vi "Screen_Traduction.vi"() -> ()   [LabVIEW 2013]
uses:
  030 - EVENTS/EnumFgvEventCommand.ctl
  ContexteTraduction.ctl
  080 - TOOLS/Traduction/Dictionnary/Dictionnaire.ctl
  080 - TOOLS/Traduction/Dictionnary/CleValeur.ctl
  090 - ERRORS/Ctrls/enumLogAndView.ctl
  080 - TOOLS/Traduction/Dictionnary/EnumCommandDictionnaire.ctl
  <vilib>/Utility/miscctls.llb/LVComboBoxStrsAndValuesArrayTypeDef.ctl
  050 - CONFIG/00 - ApplicationConfig/Ctrls/EnumFgvConfigCommand.ctl
  enumScreen.ctl
panel:
  in  "Dictionnaire":string(combo)
  in  "Supprimer Dictionnaire":bool
  in  "Dupliquer Dictionnaire":bool
  in  "Dictionnaire verrouillé ?":bool
  in  "Clés":i32[](listbox)
  in  "Supprimer Lignes":bool
  out "Valeur de référence":string
  in  "Valeur traduite":string
  in  "Bouton menu principal":bool
  # "Attention : Si la \"valeur traduite\" contient des caractères de type %s, %d, %f ..., il s'agit de caractères de formattage\nde messages dynamiques. Il faut absolument que ces caractères apparaîssent dans la chaîne modifiée, et dans\nle même ordre.\nPour info : %s remplace une chaîne de caractères, %d remplace un entier, %f remplace un nombre à virgules \nflottantes. (Voir syntaxe du langage C)"
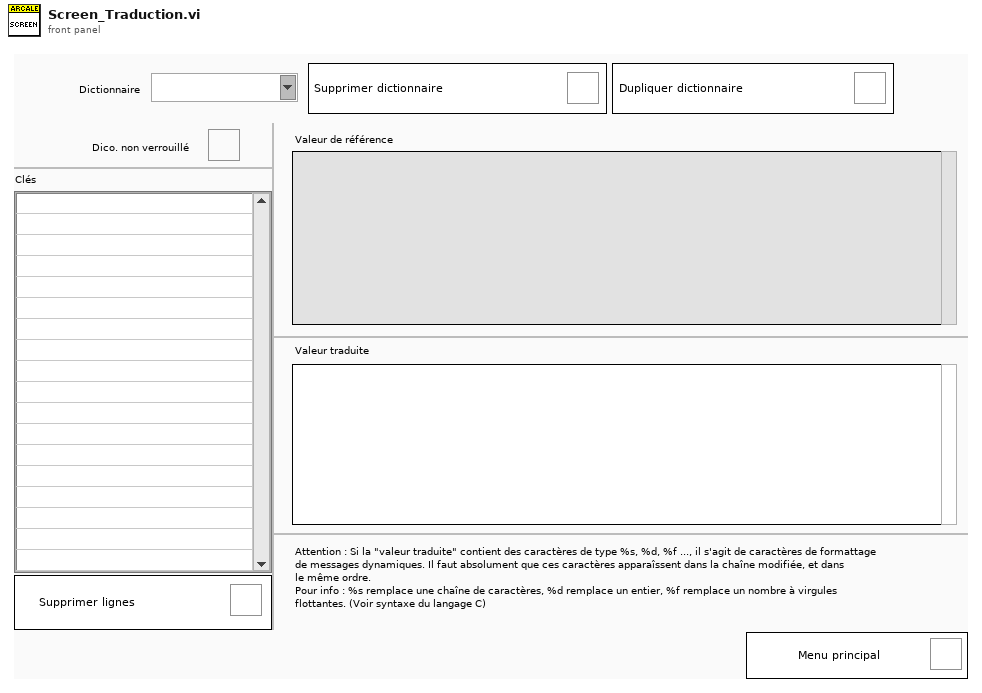
[diagram p1: front panel]
types:
  T1 = typedef "enumLogAndView.ctl" = enum16{"Log only", "Log and view"}
  T2 = typedef "ContexteTraduction.ctl" = cluster{"Dictionnaire":T3}
  T3 = typedef "Dictionnaire.ctl" = cluster{"FichierDictionnaire":path, "TabCleValeur":T4[], "DictionnaireModifié?":bool, "Traduction à réaliser ?":bool, "Interdire l'ajout de nouvelles clés ?":bool}
  T4 = typedef "CleValeur.ctl" = cluster{"Clé":string, "Valeur":string}
  T5 = typedef "EnumFgvEventCommand.ctl" = enum16{"Setup", "Cleanup", "Get"}
  T6 = typedef "EnumFgvConfigCommand.ctl" = enum16{"Load", "Get", "Set", "Save To Disk"}
  T7 = typedef "LVComboBoxStrsAndValuesArrayTypeDef.ctl" = cluster{"String":string, "Value":string}[]
  T8 = typedef "EnumCommandDictionnaire.ctl" = enum16{"Load", "Translate", "Save", "GetDico", "Set : A traduire = Vrai", "Set : A Traduire = Faux", "SetDico"}
  T9 = typedef "ApplicationConfig.ctl" = cluster{"Data Path":path, "MessageHandlerConfig":T10, "Simulation":bool, "Dictionnary":string}
  T10 = typedef "MessageHandlerConfig.ctl" = cluster{"Max log files":u32, "Max messages per file":u32}
  T11 = enum8{"Enabled", "Disabled", "Disabled and Grayed Out"}
  T12 = typedef "enumScreen.ctl" = enum16{"Test screen", "Ecran principal", "LOG", "Setup", "Popup : About", "Popup : View last message", "Popup : WebBrowser help", "Traduction", "Popup : DEBUG Process"}
  T13 = typedef "ToScreensCommand.ctl" = enum16{"Stop screen", "Stop all screens"}
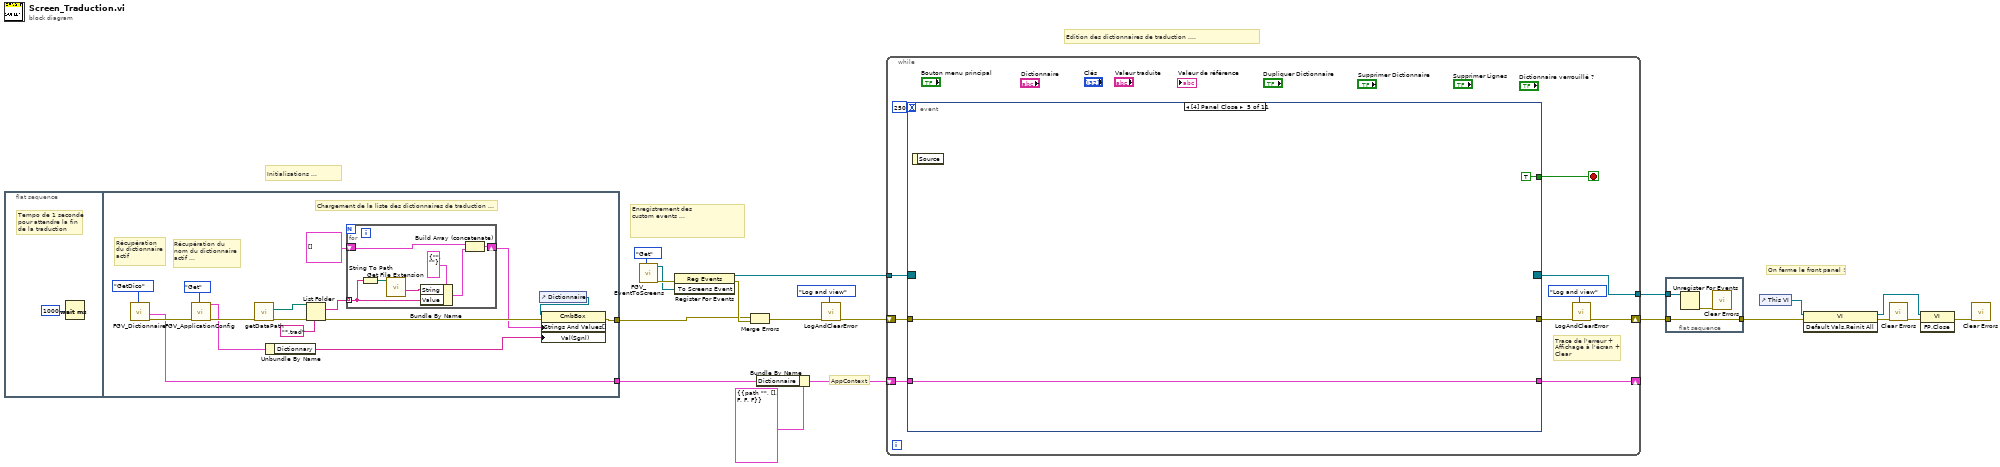
[diagram p0: block diagram]
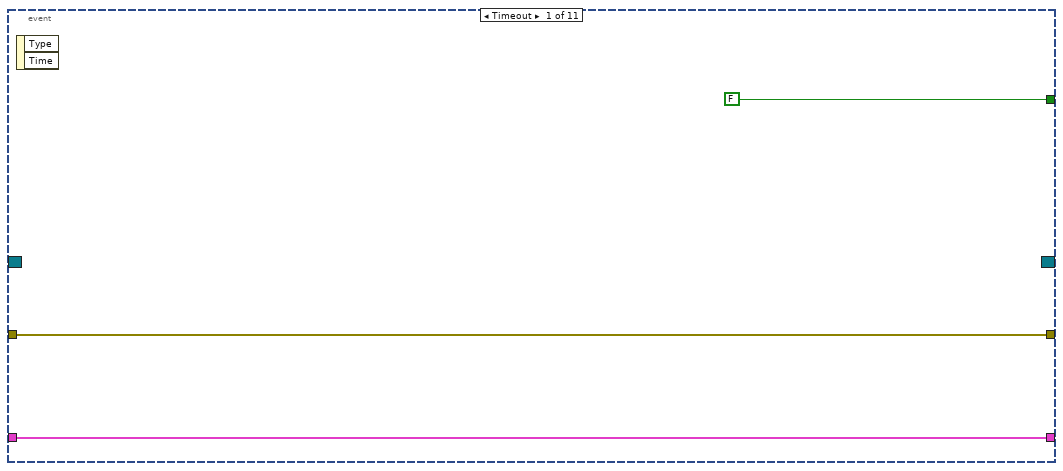
[diagram p2: hidden frame]
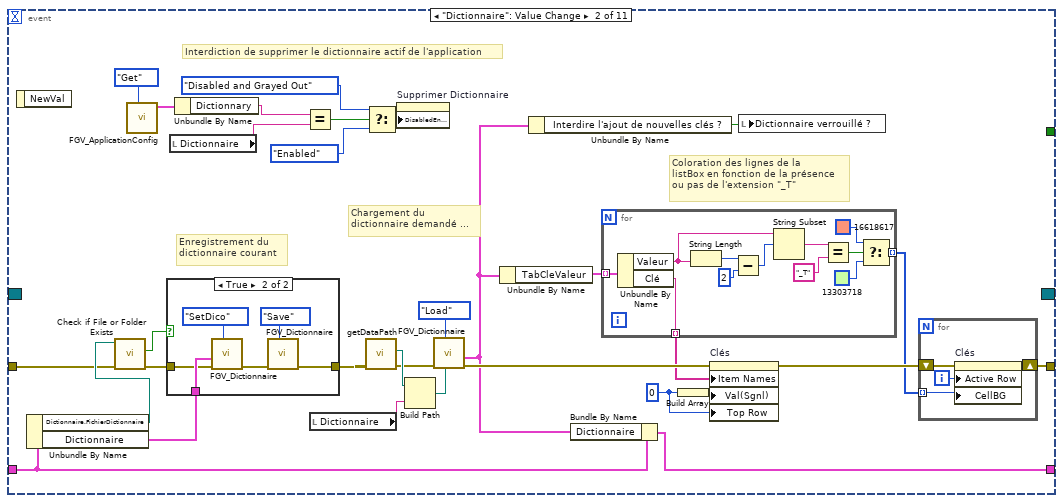
[diagram p3: hidden frame]
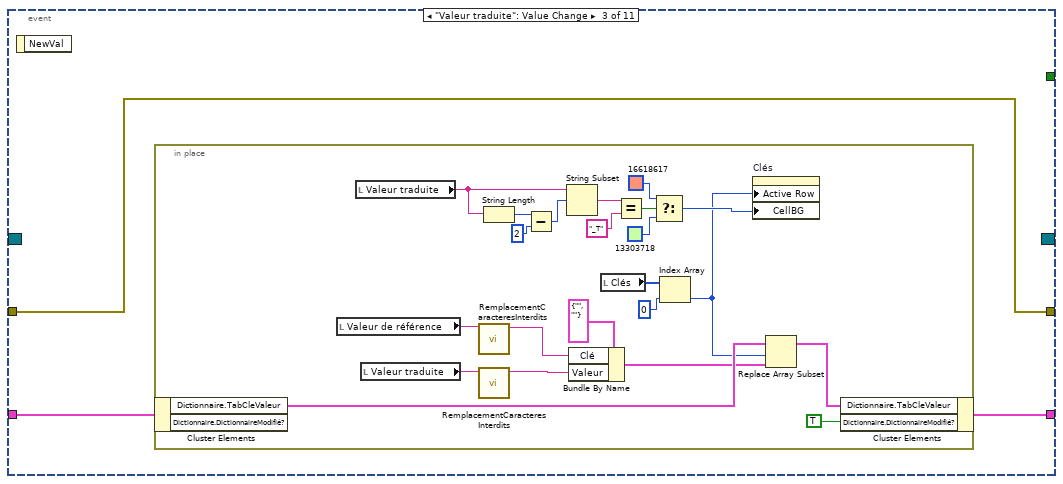
[diagram p5: hidden frame]
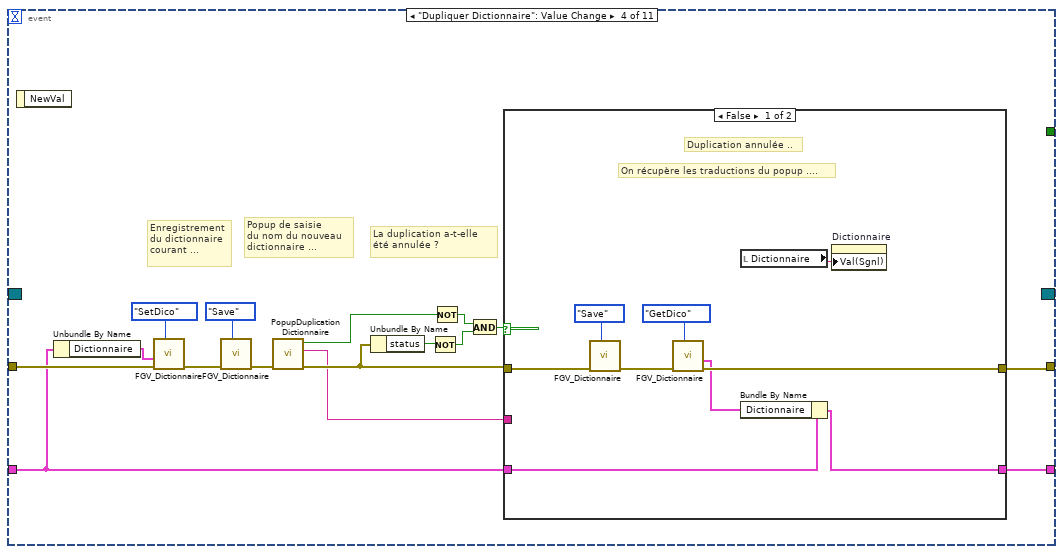
[diagram p6: hidden frame]
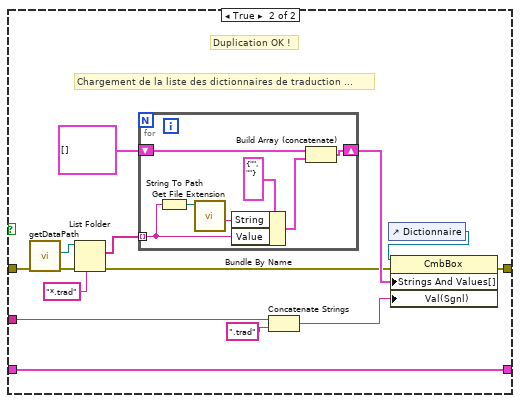
[diagram p7: hidden frame]
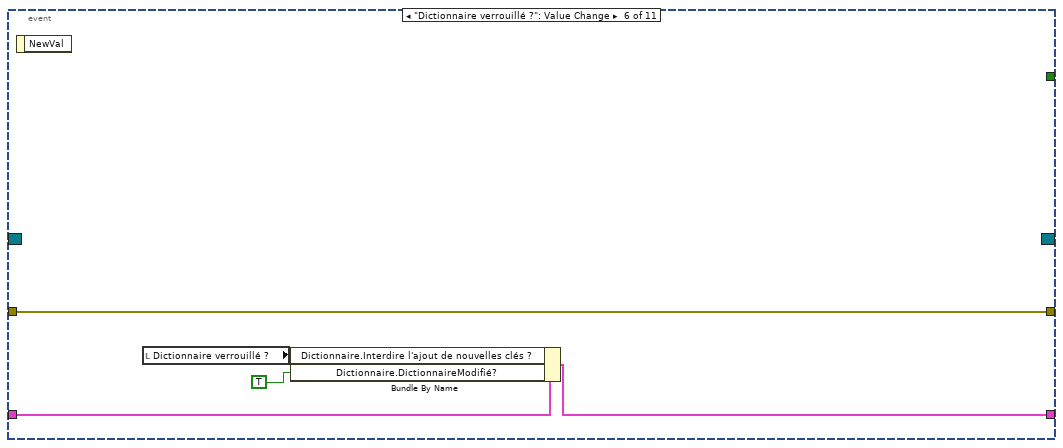
[diagram p8: hidden frame]
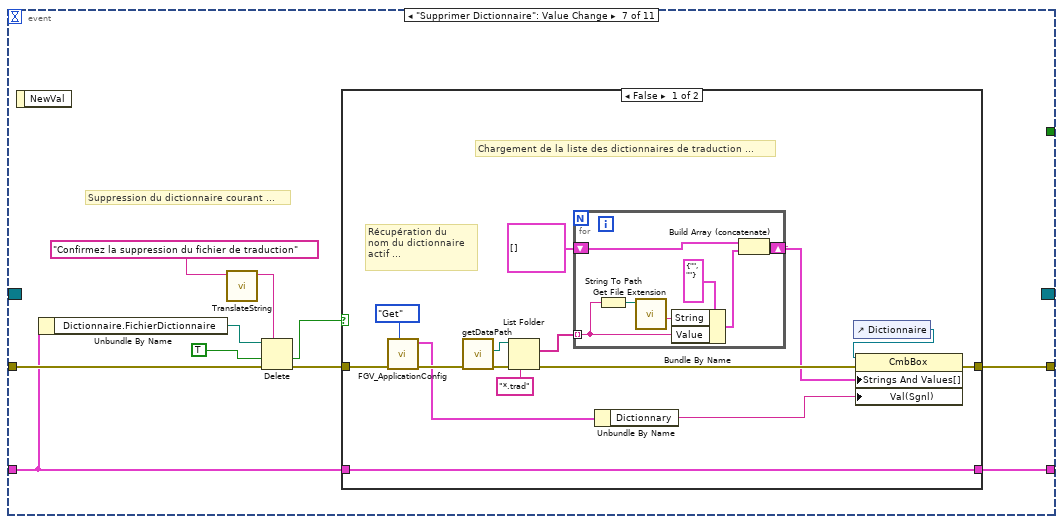
[diagram p9: hidden frame]
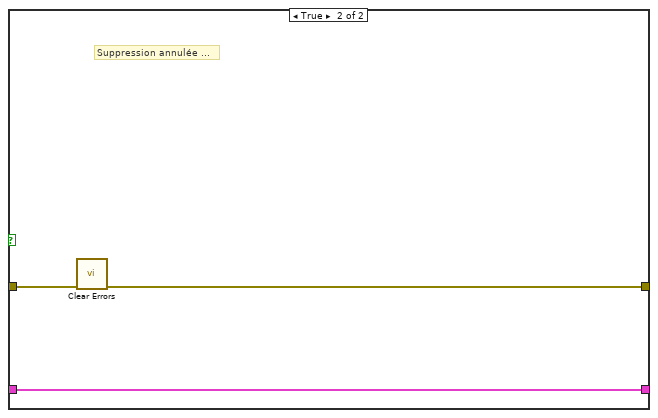
[diagram p10: hidden frame]
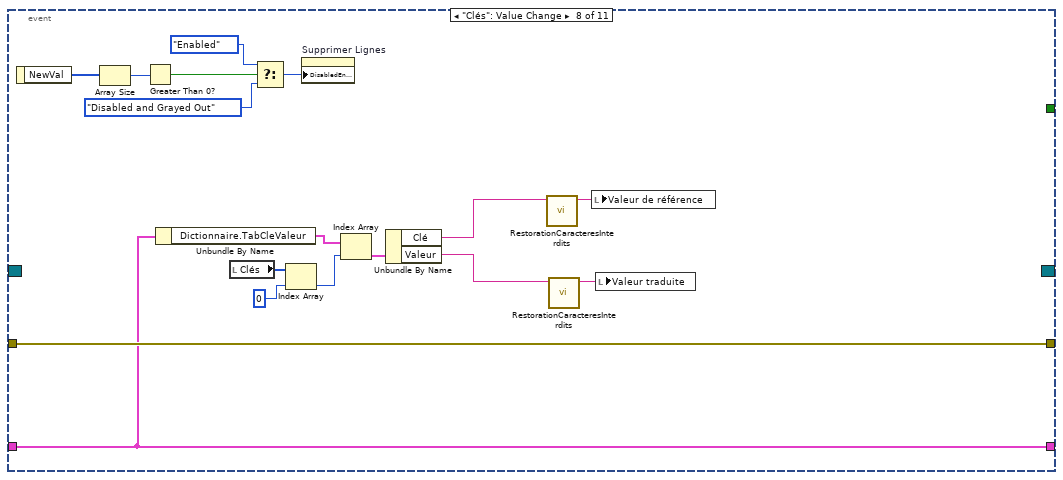
[diagram p11: hidden frame]
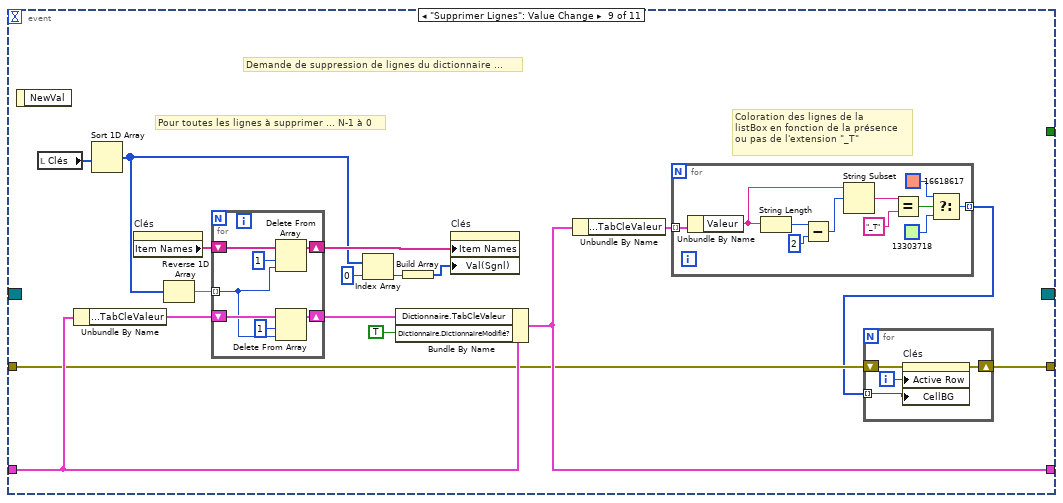
[diagram p12: hidden frame]
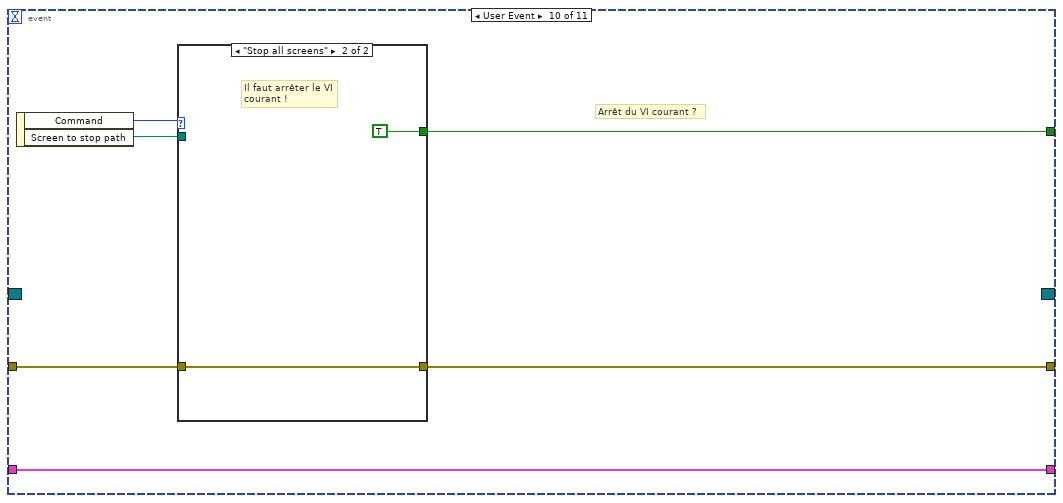
[diagram p13: hidden frame]
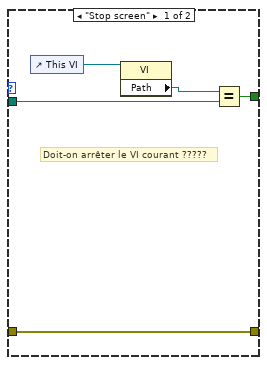
[diagram p14: hidden frame]
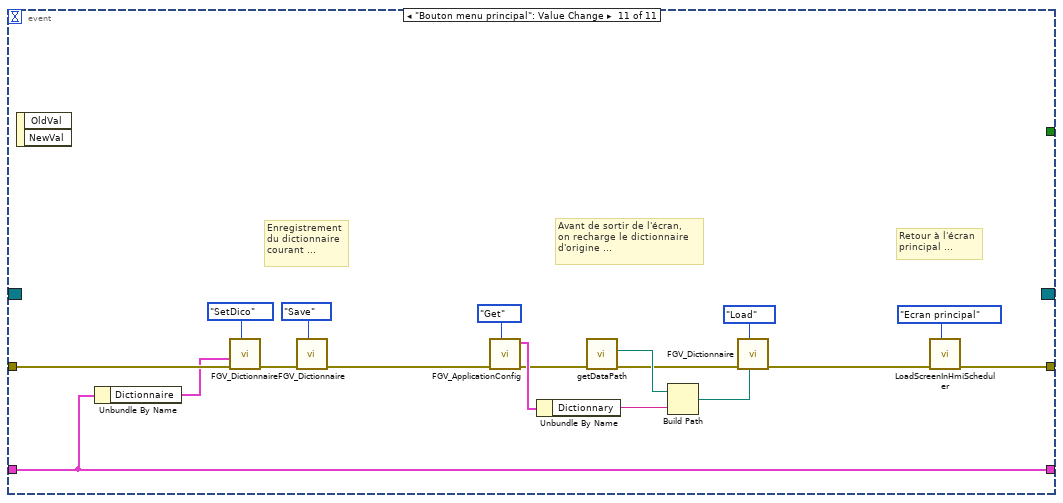
[diagram p15: hidden frame]
diagram:
  # "AppContext"
  # "Enregistrement des\ncustom events ..."
  # "Initialisations ..."
  # "On ferme le front panel !"
  # "Edition des dictionnaires de traduction ...."
  n1 = flat-sequence {
    tunnel: [w29] -> w9
    tunnel: [w22] -> w7
    frame #0 {
      # "Tempo de 1 seconde\npour attendre la fin\nde la traduction"
      n2 = Wait (ms)(milliseconds to wait=u32 1000) -> ()  [unwired: 1 out]
    }
    frame #1 {
      # "Récupération du\nnom du dictionnaire\nactif ..."
      # "Chargement de la liste des dictionnaires de traduction ..."
      # "Récupération \ndu dictionnaire\nactif"
      n3 = call "FGV_Dictionnaire.vi"("Command"=EnumCommandDictionnaire."GetDico") -> ("error out"=w28:errorcluster, "Dictionnaire Out"=w22:T3)  [unwired: 8 in, 1 out]
      n4 = call "FGV_ApplicationConfig.vi"("Command"=EnumFgvConfigCommand."Get", "error in (no error)"=w28) -> ("error out"=w27:errorcluster, "ApplicationConfigOut"=w25:T9)  [unwired: 8 in]
      n5 = call "getDataPath.vi"("error in (no error)"=w27) -> ("error out"=w32:errorcluster, "DataPath"=w36:path)  [unwired: 9 in]
      n6 = Unbundle By Name(w25) -> ("Dictionnary"=w24:string)
      n7 = List Folder(path=w36, pattern="*.trad", error in=w32) -> (filenames=w34:string[], error out=w31:errorcluster)  [unwired: 1 in, 2 out]
      n8 = for {
        tunnel: w34 -> [w40] mode=indexing
        shift-right: [w43] -> w23
        shift-left: T7 [] ("Strings And Values []") -> [w44]
        n9 = String To Path(string=w40) -> (path=w39:path)
        n10 = call <vilib>:"Get File Extension.vi"("file"=w39) -> ("filename without extension"=w38:string)  [unwired: 7 in, 3 out]
        n11 = Bundle By Name(cluster=cluster{"String":string, "Value":string} {"String"="", "Value"=""}, "String"=w38, "Value"=w40) -> (w41:cluster{"String":string, "Value":string})
        n12 = Build Array (concatenate)(w44, w41) -> (w43:T7)
      }
      n13 = control-ref of="Dictionnaire"() -> (w30:refnum<vi>)
      n14 = property on="Property Node" class="CmbBox"(reference=w30, error in=w31, "Strings And Values[]"=w23, "Val(Sgnl)"=w24) -> (error out=w29:errorcluster)  [unwired: 1 out]
    }
  }
  n15 = call "FGV_EventToScreens.vi"("Command"=EnumFgvEventCommand."Get") -> ("error out"=w20:errorcluster, "To Screens Event"=w19:refnum<user-event>)  [unwired: 9 in]
  n16 = register-events(error in=w20, w19) -> (reference out=w18:refnum<event-registration>, error out=w11:errorcluster)  [unwired: 1 in]
  n17 = Merge Errors(w9, w11) -> (w5:errorcluster)
  n18 = Bundle By Name(cluster=T2 {"Dictionnaire"={"FichierDictionnaire"=path "", "TabCleValeur"=[], "DictionnaireModifié?"=FALSE, "Traduction à réaliser ?"=FALSE, "Interdire l'ajout de nouvelles clés ?"=FALSE}} ("Contexte"), "Dictionnaire"=w7) -> (w8:T2)
  n19 = call "LogAndClearError.vi"("Log and view ?"=enumLogAndView."Log and view", "error in (no error)"=w5) -> ("error out"=w4:errorcluster)  [unwired: 9 in]
  n20 = while {
    tunnel: w18 -> [w54]
    shift-right: [w48] -> w16
    shift-left: w4 -> [w53]
    tunnel: [w52] -> w17
    shift-right: [w49] -> _
    shift-left: w8 -> [w50]
    stop <- w51 stop-if-true
    # "Trace de l'erreur +\nAffichage à l'écran +\nClear"
    n21 = event shown="[4] Panel Close" {
      selector: w54 -> [_ _ _ _ _ _ _ _ _ _ _]
      dyn-events: [_ _ _ _ _ _ _ _ _ _ _] -> w52
      timeout: 250 -> [_ _ _ _ _ _ _ _ _ _ _]
      tunnel: w53 -> [w57 w68 w112 w149 w185 w190 w200 w240 w245 w286 w298]
      tunnel: [w57 w78 w112 w140 w185 w190 w192 w240 w244 w285 w311] -> w47
      tunnel: [FALSE _ _ _ TRUE _ _ _ _ w283 _] -> w51
      tunnel: w50 -> [w55 w75 w114 w138 w184 w189 w193 w239 w256 w282 w296]
      tunnel: [w55 w82 w113 w137 w184 w188 w191 w239 w246 w282 w296] -> w49
      event Timeout {
        n22 = event-data() -> ()  [unwired: 1 in, 2 out]
      }
      event "Dictionnaire": Value Change {
        w71 = 0 ("Value (Signaling)")
        # "Interdiction de supprimer le dictionnaire actif de l'application"
        # "Coloration des lignes de la\nlistBox en fonction de la présence\nou pas de l'extension \"_T\""
        # "Enregistrement du\ndictionnaire courant"
        # "Chargement du \ndictionnaire demandé ..."
        n23 = event-data() -> ()  [unwired: 1 in, 1 out]
        n24 = Unbundle By Name(w75) -> ("Dictionnaire.FichierDictionnaire"=w73:path, "Dictionnaire"=w76:T3)
        n25 = call <vilib>:"Check if File or Folder Exists.vi"("error in (no error)"=w68, "path"=w73) -> ("error out"=w74:errorcluster, "file or folder exists?"=w72:bool)  [unwired: 7 in, 1 out]
        n26 = call "FGV_ApplicationConfig.vi"("Command"=EnumFgvConfigCommand."Get") -> ("ApplicationConfigOut"=w66:T9)  [unwired: 9 in, 1 out]
        n27 = case shown="True" w72 {
          tunnel: [w89 w94] -> w81
          tunnel: w76 -> [_ w91]
          tunnel: w74 -> [w89 w90]
          frame False {
          }
          frame True {
            n28 = call "FGV_Dictionnaire.vi"("Command"=EnumCommandDictionnaire."SetDico", "error in (no error)"=w90, "Dictionnaire In"=w91) -> ("error out"=w92:errorcluster)  [unwired: 6 in, 2 out]
            n29 = call "FGV_Dictionnaire.vi"("Command"=EnumCommandDictionnaire."Save", "error in (no error)"=w92) -> ("error out"=w94:errorcluster)  [unwired: 7 in, 2 out]
          }
        }
        n30 = local read "Dictionnaire"() -> (w65:string)
        n31 = Unbundle By Name(w66) -> ("Dictionnary"=w64:string)
        n32 = Equal?(x=w64, y=w65) -> (x = y?=w61:bool)
        n33 = local read "Dictionnaire"() -> (w77:string)
        n34 = call "getDataPath.vi"("error in (no error)"=w81) -> ("error out"=w86:errorcluster, "DataPath"=w88:path)  [unwired: 9 in]
        n35 = Select(t=T11."Disabled and Grayed Out" ("Disabled"), s=w61, f=T11."Enabled" ("Disabled")) -> (s? t:f=w63:T11)
        n36 = property on="Supprimer Dictionnaire" class="Bool"("DisabledEnum"=w63) -> ()  [unwired: 2 in, 2 out]
        n37 = Build Path(base path=w88, name or relative path=w77) -> (appended path=w85:path)
        n38 = call "FGV_Dictionnaire.vi"("FichierDictionnaire"=w85, "Command"=EnumCommandDictionnaire."Load", "error in (no error)"=w86) -> ("error out"=w84:errorcluster, "Dictionnaire Out"=w59:T3)  [unwired: 6 in, 1 out]
        n39 = Unbundle By Name(w59) -> ("TabCleValeur"=w69:T4[])
        n40 = Unbundle By Name(w59) -> ("Interdire l'ajout de nouvelles clés ?"=w58:bool)
        n41 = Bundle By Name(cluster=w75, "Dictionnaire"=w59) -> (w82:T2)
        n42 = for {
          tunnel: w69 -> [w111] mode=indexing
          tunnel: [w110] -> w83 mode=indexing
          tunnel: [w100] -> w79 mode=indexing
          n43 = Unbundle By Name(w111) -> ("Valeur"=w109:string, "Clé"=w110:string)
          n44 = String Length(string=w109) -> (length=w108:i32)
          n45 = Subtract(x=w108, y=2) -> (x-y=w106:i32)
          n46 = String Subset(string=w109, offset (0)=w106) -> (substring=w105:string)  [unwired: 1 in]
          n47 = Equal?(x=w105, y="_T") -> (x = y?=w103:bool)
          n48 = Select(t=u32 16618617, s=w103, f=u32 13303718) -> (s? t:f=w100:u32)
        }
        n49 = Build Array(w71) -> (w70:i32[])
        n50 = property on="Clés" class="LstBox (strict)"(error in=w84, "Item Names"=w83, "Val(Sgnl)"=w70, "Top Row"=w71) -> (error out=w80:errorcluster)  [unwired: 1 in, 1 out]
        n51 = local write "Dictionnaire verrouillé ?"(w58) -> ()
        n52 = for {
          shift-right: [w98] -> w78
          shift-left: w80 -> [w99]
          tunnel: w79 -> [w97] mode=indexing
          i -> [w96]
          n53 = property on="Clés" class="LstBox (strict)"(error in=w99, "Active Row"=w96, "CellBG"=w97) -> (error out=w98:errorcluster)  [unwired: 1 in, 1 out]
        }
      }
      event "Valeur traduite": Value Change {
        n54 = event-data() -> ()  [unwired: 1 in, 1 out]
        n55 = in-place {
          n56 = in-place-cluster #1(w114) -> ("Dictionnaire.TabCleValeur"=w135:T4[])  [unwired: 1 out]
          n57 = local read "Valeur de référence"() -> (w121:string)
          n58 = local read "Valeur traduite"() -> (w123:string)
          n59 = local read "Valeur traduite"() -> (w119:string)
          n60 = call "RemplacementCaracteresInterdits.vi"("String In"=w121) -> ("String Out"=w120:string)  [unwired: 9 in, 1 out]
          n61 = call "RemplacementCaracteresInterdits.vi"("String In"=w119) -> ("String Out"=w118:string)  [unwired: 9 in, 1 out]
          n62 = String Length(string=w123) -> (length=w131:i32)
          n63 = Subtract(x=w131, y=2) -> (x-y=w129:i32)
          n64 = String Subset(string=w123, offset (0)=w129) -> (substring=w128:string)  [unwired: 1 in]
          n65 = Bundle By Name(cluster=T4 {"Clé"="", "Valeur"=""} ("new element/subarray"), "Clé"=w120, "Valeur"=w118) -> (w132:T4)
          n66 = local read "Clés"() -> (w117:i32[])
          n67 = Equal?(x=w128, y="_T") -> (x = y?=w126:bool)
          n68 = Select(t=u32 16618617, s=w126, f=u32 13303718) -> (s? t:f=w122:u32)
          n69 = Index Array(array=w117, index=0) -> (element=w115:i32)
          n70 = property on="Clés" class="LstBox (strict)"("Active Row"=w115, "CellBG"=w122) -> ()  [unwired: 2 in, 2 out]
          n71 = Replace Array Subset(array=w135, new element=w132, index=w115) -> (w134:T4[])
          n72 = in-place-cluster #1("Dictionnaire.TabCleValeur"=w134, "Dictionnaire.DictionnaireModifié?"=TRUE) -> (w113:T2)
        }
      }
      event "Dupliquer Dictionnaire": Value Change {
        # "La duplication a-t-elle\nété annulée ?"
        # "Popup de saisie\ndu nom du nouveau\ndictionnaire ..."
        # "Enregistrement\ndu dictionnaire\ncourant ..."
        n73 = event-data() -> ()  [unwired: 1 in, 1 out]
        n74 = Unbundle By Name(w138) -> ("Dictionnaire"=w147:T3)
        n75 = call "FGV_Dictionnaire.vi"("Command"=EnumCommandDictionnaire."SetDico", "error in (no error)"=w149, "Dictionnaire In"=w147) -> ("error out"=w150:errorcluster)  [unwired: 6 in, 2 out]
        n76 = call "FGV_Dictionnaire.vi"("Command"=EnumCommandDictionnaire."Save", "error in (no error)"=w150) -> ("error out"=w148:errorcluster)  [unwired: 7 in, 2 out]
        n77 = call "PopupDuplicationDictionnaire.vi"("error in (no error)"=w148) -> ("error out"=w141:errorcluster, "Nouveau dictionnaire Out"=w139:string, "Edition annulée ?"=w146:bool)  [unwired: 8 in]
        n78 = Unbundle By Name(w141) -> ("status"=w145:bool)
        n79 = Not(x=w145) -> (.not. x?=w143:bool)
        n80 = Not(x=w146) -> (.not. x?=w144:bool)
        n81 = And(x=w144, y=w143) -> (x .and. y?=w142:bool)
        n82 = case shown="False" w142 {
          tunnel: w141 -> [w160 w167]
          tunnel: [w157 w166] -> w140
          tunnel: w139 -> [_ w165]
          tunnel: w138 -> [w156 w162]
          tunnel: [w155 w162] -> w137
          frame False {
            # "On récupère les traductions du popup ...."
            # "Duplication annulée .."
            n83 = call "FGV_Dictionnaire.vi"("Command"=EnumCommandDictionnaire."Save", "error in (no error)"=w160) -> ("error out"=w158:errorcluster)  [unwired: 7 in, 2 out]
            n84 = call "FGV_Dictionnaire.vi"("Command"=EnumCommandDictionnaire."GetDico", "error in (no error)"=w158) -> ("error out"=w157:errorcluster, "Dictionnaire Out"=w154:T3)  [unwired: 7 in, 1 out]
            n85 = local read "Dictionnaire"() -> (w153:string)
            n86 = Bundle By Name(cluster=w156, "Dictionnaire"=w154) -> (w155:T2)
            n87 = property on="Dictionnaire" class="CmbBox"("Val(Sgnl)"=w153) -> ()  [unwired: 2 in, 2 out]
          }
          frame True {
            # "Chargement de la liste des dictionnaires de traduction ..."
            # "Duplication OK !"
            n88 = call "getDataPath.vi"("error in (no error)"=w167) -> ("error out"=w170:errorcluster, "DataPath"=w175:path)  [unwired: 9 in]
            n89 = List Folder(path=w175, pattern="*.trad", error in=w170) -> (filenames=w173:string[], error out=w169:errorcluster)  [unwired: 1 in, 2 out]
            n90 = for {
              tunnel: w173 -> [w176] mode=indexing
              shift-right: [w181] -> w171
              shift-left: T7 [] ("Strings And Values []") -> [w182]
              n91 = String To Path(string=w176) -> (path=w178:path)
              n92 = call <vilib>:"Get File Extension.vi"("file"=w178) -> ("filename without extension"=w177:string)  [unwired: 7 in, 3 out]
              n93 = Bundle By Name(cluster=cluster{"String":string, "Value":string} {"String"="", "Value"=""}, "String"=w177, "Value"=w176) -> (w179:cluster{"String":string, "Value":string})
              n94 = Build Array (concatenate)(w182, w179) -> (w181:T7)
            }
            n95 = Concatenate Strings(w165, ".trad" ("string")) -> (w164:string)
            n96 = control-ref of="Dictionnaire"() -> (w168:refnum<vi>)
            n97 = property on="Property Node" class="CmbBox"(reference=w168, error in=w169, "Strings And Values[]"=w171, "Val(Sgnl)"=w164) -> (error out=w166:errorcluster)  [unwired: 1 out]
          }
        }
      }
      event Panel Close {
        n98 = event-data() -> ()  [unwired: 1 in, 1 out]
      }
      event "Dictionnaire verrouillé ?": Value Change {
        n99 = event-data() -> ()  [unwired: 1 in, 1 out]
        n100 = local read "Dictionnaire verrouillé ?"() -> (w187:bool)
        n101 = Bundle By Name(cluster=w189, "Dictionnaire.Interdire l'ajout de nouvelles clés ?"=w187, "Dictionnaire.DictionnaireModifié?"=TRUE) -> (w188:T2)
      }
      event "Supprimer Dictionnaire": Value Change {
        # "Suppression du dictionnaire courant ..."
        n102 = event-data() -> ()  [unwired: 1 in, 1 out]
        n103 = Unbundle By Name(w193) -> ("Dictionnaire.FichierDictionnaire"=w199:path)
        n104 = call "TranslateString.vi"("String"="Confirmez la suppression du fichier de traduction") -> ("Translated String"=w197:string)  [unwired: 9 in, 1 out]
        n105 = Delete(prompt (Delete)=w197, path (use dialog)=w199, confirm (F)=TRUE, error in=w200) -> (cancelled=w195:bool, error out=w194:errorcluster)  [unwired: 1 in, 1 out]
        n106 = case shown="False" w195 {
          tunnel: w194 -> [w204 w225]
          tunnel: w193 -> [w206 w224]
          tunnel: [w207 w223] -> w192
          tunnel: [w206 w224] -> w191
          frame False {
            # "Récupération du\nnom du dictionnaire\nactif ..."
            # "Chargement de la liste des dictionnaires de traduction ..."
            n107 = call "FGV_ApplicationConfig.vi"("Command"=EnumFgvConfigCommand."Get", "error in (no error)"=w204) -> ("error out"=w203:errorcluster, "ApplicationConfigOut"=w202:T9)  [unwired: 8 in]
            n108 = call "getDataPath.vi"("error in (no error)"=w203) -> ("error out"=w211:errorcluster, "DataPath"=w215:path)  [unwired: 9 in]
            n109 = List Folder(path=w215, pattern="*.trad", error in=w211) -> (filenames=w213:string[], error out=w210:errorcluster)  [unwired: 1 in, 2 out]
            n110 = for {
              tunnel: w213 -> [w218] mode=indexing
              shift-right: [w221] -> w208
              shift-left: T7 [] ("Strings And Values []") -> [w222]
              n111 = String To Path(string=w218) -> (path=w217:path)
              n112 = call <vilib>:"Get File Extension.vi"("file"=w217) -> ("filename without extension"=w216:string)  [unwired: 7 in, 3 out]
              n113 = Bundle By Name(cluster=cluster{"String":string, "Value":string} {"String"="", "Value"=""}, "String"=w216, "Value"=w218) -> (w219:cluster{"String":string, "Value":string})
              n114 = Build Array (concatenate)(w222, w219) -> (w221:T7)
            }
            n115 = Unbundle By Name(w202) -> ("Dictionnary"=w201:string)
            n116 = control-ref of="Dictionnaire"() -> (w209:refnum<vi>)
            n117 = property on="Property Node" class="CmbBox"(reference=w209, error in=w210, "Strings And Values[]"=w208, "Val(Sgnl)"=w201) -> (error out=w207:errorcluster)  [unwired: 1 out]
          }
          frame True {
            # "Suppression annulée ..."
            n118 = call <vilib>:"Clear Errors.vi"("error in (no error)"=w225) -> ("error out"=w223:errorcluster)  [unwired: 6 in]
          }
        }
      }
      event "Clés": Value Change {
        n119 = event-data() -> ("NewVal"=w231:i32[])  [unwired: 1 in]
        n120 = Array Size(array=w231) -> (size(s)=w230:i32)
        n121 = Greater Than 0?(x=w230) -> (x > 0?=w229:bool)
        n122 = Unbundle By Name(w239) -> ("Dictionnaire.TabCleValeur"=w242:T4[])
        n123 = local read "Clés"() -> (w234:i32[])
        n124 = Select(t=T11."Enabled" ("Disabled"), s=w229, f=T11."Disabled and Grayed Out" ("Disabled")) -> (s? t:f=w228:T11)
        n125 = Index Array(array=w234, index=0) -> (element=w232:i32)
        n126 = property on="Supprimer Lignes" class="Bool"("DisabledEnum"=w228) -> ()  [unwired: 2 in, 2 out]
        n127 = Index Array(array=w242, index=w232) -> (element=w241:T4)
        n128 = Unbundle By Name(w241) -> ("Clé"=w238:string, "Valeur"=w236:string)
        n129 = call "RestorationCaracteresInterdits.vi"("String In"=w238) -> ("String Out"=w237:string)  [unwired: 9 in, 1 out]
        n130 = call "RestorationCaracteresInterdits.vi"("String In"=w236) -> ("String Out"=w235:string)  [unwired: 9 in, 1 out]
        n131 = local write "Valeur de référence"(w237) -> ()
        n132 = local write "Valeur traduite"(w235) -> ()
      }
      event "Supprimer Lignes": Value Change {
        # "Coloration des lignes de la\nlistBox en fonction de la présence\nou pas de l'extension \"_T\""
        # "Pour toutes les lignes à supprimer ... N-1 à 0"
        # "Demande de suppression de lignes du dictionnaire ..."
        n133 = event-data() -> ()  [unwired: 1 in, 1 out]
        n134 = local read "Clés"() -> (w259:i32[])
        n135 = Unbundle By Name(w256) -> ("Dictionnaire.TabCleValeur"=w257:T4[])
        n136 = Sort 1D Array(array=w259) -> (sorted array=w251:i32[])
        n137 = property on="Clés" class="LstBox (strict)"() -> ("Item Names"=w254:string[])  [unwired: 2 in, 2 out]
        n138 = Reverse 1D Array(array=w251) -> (reversed array=w258:i32[])
        n139 = for {
          tunnel: w258 -> [w275] mode=indexing
          shift-right: [w279] -> w253
          shift-left: w257 -> [w281]
          shift-right: [w277] -> w252
          shift-left: w254 -> [w278]
          n140 = Delete From Array(array=w278, length=1, index=w275) -> (array with subset deleted=w277:string[])  [unwired: 1 out]
          n141 = Delete From Array(array=w281, length=1, index=w275) -> (array with subset deleted=w279:T4[])  [unwired: 1 out]
        }
        n142 = Index Array(array=w251, index=0) -> (element=w249:i32)
        n143 = Bundle By Name(cluster=w256, "Dictionnaire.TabCleValeur"=w253, "Dictionnaire.DictionnaireModifié?"=TRUE) -> (w246:T2)
        n144 = Build Array(w249) -> (w248:i32[])
        n145 = property on="Clés" class="LstBox (strict)"("Item Names"=w252, "Val(Sgnl)"=w248) -> ()  [unwired: 2 in, 2 out]
        n146 = Unbundle By Name(w246) -> ("Dictionnaire.TabCleValeur"=w247:T4[])
        n147 = for {
          tunnel: w247 -> [w274] mode=indexing
          tunnel: [w264] -> w243 mode=indexing
          n148 = Unbundle By Name(w274) -> ("Valeur"=w273:string)
          n149 = String Length(string=w273) -> (length=w272:i32)
          n150 = Subtract(x=w272, y=2) -> (x-y=w270:i32)
          n151 = String Subset(string=w273, offset (0)=w270) -> (substring=w269:string)  [unwired: 1 in]
          n152 = Equal?(x=w269, y="_T") -> (x = y?=w267:bool)
          n153 = Select(t=u32 16618617, s=w267, f=u32 13303718) -> (s? t:f=w264:u32)
        }
        n154 = for {
          shift-right: [w262] -> w244
          shift-left: w245 -> [w263]
          tunnel: w243 -> [w261] mode=indexing
          i -> [w260]
          n155 = property on="Clés" class="LstBox (strict)"(error in=w263, "Active Row"=w260, "CellBG"=w261) -> (error out=w262:errorcluster)  [unwired: 1 in, 1 out]
        }
      }
      event User Event {
        # "Arrêt du VI courant ?"
        n156 = event-data() -> ("Command"=w287:T13, "Screen to stop path"=w284:path)  [unwired: 1 in]
        n157 = case shown="\"Stop all screens\"" w287 {
          tunnel: w286 -> [w292 w293]
          tunnel: [w292 w293] -> w285
          tunnel: w284 -> [w289 _]
          tunnel: [w288 TRUE] -> w283
          frame "Stop screen" {
            # "Doit-on arrêter le VI courant ?????"
            n158 = control-ref of="This VI"() -> (w291:refnum<vi>)
            n159 = property class="VI"(reference=w291) -> ("Path"=w290:path)  [unwired: 1 in, 2 out]
            n160 = Equal?(x=w290, y=w289) -> (x = y?=w288:bool)
          }
          frame "Stop all screens" {
            # "Il faut arrêter le VI\ncourant !"
          }
        }
      }
      event "Bouton menu principal": Value Change {
        # "Retour à l'écran\nprincipal ..."
        # "Enregistrement\ndu dictionnaire\ncourant ..."
        # "Avant de sortir de l'écran, \non recharge le dictionnaire \nd'origine ..."
        n161 = event-data() -> ()  [unwired: 1 in, 2 out]
        n162 = Unbundle By Name(w296) -> ("Dictionnaire"=w295:T3)
        n163 = call "FGV_Dictionnaire.vi"("Command"=EnumCommandDictionnaire."SetDico", "error in (no error)"=w298, "Dictionnaire In"=w295) -> ("error out"=w297:errorcluster)  [unwired: 6 in, 2 out]
        n164 = call "FGV_Dictionnaire.vi"("Command"=EnumCommandDictionnaire."Save", "error in (no error)"=w297) -> ("error out"=w307:errorcluster)  [unwired: 7 in, 2 out]
        n165 = call "FGV_ApplicationConfig.vi"("Command"=EnumFgvConfigCommand."Get", "error in (no error)"=w307) -> ("error out"=w305:errorcluster, "ApplicationConfigOut"=w306:T9)  [unwired: 8 in]
        n166 = Unbundle By Name(w306) -> ("Dictionnary"=w303:string)
        n167 = call "getDataPath.vi"("error in (no error)"=w305) -> ("error out"=w302:errorcluster, "DataPath"=w304:path)  [unwired: 9 in]
        n168 = Build Path(base path=w304, name or relative path=w303) -> (appended path=w300:path)
        n169 = call "FGV_Dictionnaire.vi"("FichierDictionnaire"=w300, "Command"=EnumCommandDictionnaire."Load", "error in (no error)"=w302) -> ("error out"=w301:errorcluster)  [unwired: 6 in, 2 out]
        n170 = call "LoadScreenInHmiScheduler.vi"("Enum Screen"=enumScreen."Ecran principal", "error in (no error)"=w301) -> ("error out"=w311:errorcluster)  [unwired: 9 in]
      }
    }
    n171 = call "LogAndClearError.vi"("Log and view ?"=enumLogAndView."Log and view", "error in (no error)"=w47) -> ("error out"=w48:errorcluster)  [unwired: 9 in]
  }
  n172 = flat-sequence {
    tunnel: w17 -> [w315]
    tunnel: w16 -> [w313]
    tunnel: [w313] -> w14
    frame #0 {
      n173 = Unregister For Events(event registration refnum=w315) -> (error out=w314:errorcluster)  [unwired: 1 in]
      n174 = call <vilib>:"Clear Errors.vi"("error in (no error)"=w314) -> ()  [unwired: 6 in, 1 out]
    }
  }
  n175 = control-ref of="This VI"() -> (w13:refnum<vi>)
  n176 = invoke class="VI" method="Default Vals.Reinit All"(reference=w13, error in=w14) -> (reference out=w1:refnum<vi>, error out=w15:errorcluster)  [unwired: 1 in, 1 out]
  n177 = call <vilib>:"Clear Errors.vi"("error in (no error)"=w15) -> ("error out"=w2:errorcluster)  [unwired: 6 in]
  n178 = invoke class="VI" method="FP.Close"(reference=w1, error in=w2) -> (error out=w3:errorcluster)  [unwired: 1 in, 2 out]
  n179 = call <vilib>:"Clear Errors.vi"("error in (no error)"=w3) -> ()  [unwired: 6 in, 1 out]
